vi "Configure Setting Value.vi"(8 "error in (no error)":errorcluster, 9 "Setting Value (0)":dbl min=0.0 step=0.1 format="%^#_6g", 10 "Operation Mode (0: Current)":u16(ring) items=["Current", "Voltage", "Resistance", "Power"], 11 "VISA resource name":refnum<visa-resource-name>) -> (0 "error out":errorcluster, 3 "VISA resource name out":refnum<visa-resource-name>)   [LabVIEW 2021, in "HH PLI Series.lvlib"]
doc: "Sets the operation mode and a static value corresponding to the selected operation mode."
uses:
  HH PLI Series.lvlib
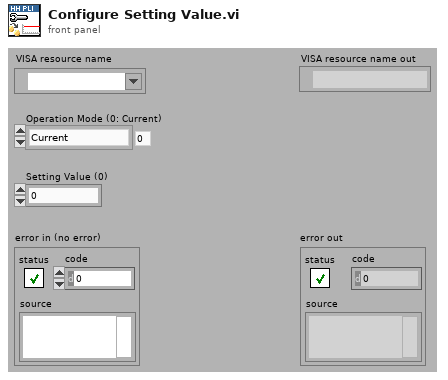
[diagram p1: front panel]
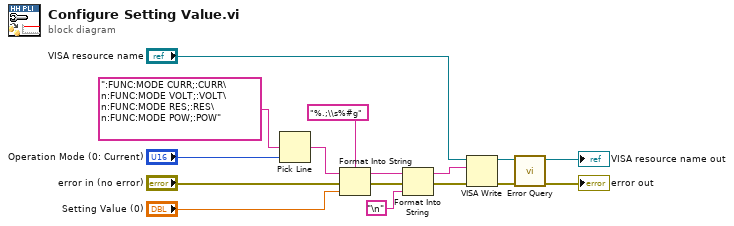
[diagram p0: block diagram]
diagram:
  n1 = Pick Line(multi-line string=":FUNC:MODE CURR;:CURR\n:FUNC:MODE VOLT;:VOLT\n:FUNC:MODE RES;:RES\n:FUNC:MODE POW;:POW", line index="Operation Mode (0: Current)") -> (output string=w6:string)  [unwired: 1 in]
  n2 = Format Into String(format string="%.;\\s%#g", initial string=w6, error in="error in (no error)", "Setting Value (0)") -> (resulting string=w5:string, error out=w2:errorcluster)
  n3 = Format Into String(initial string=w5, error in=w2, "\n") -> (resulting string=w1:string, error out=w4:errorcluster)  [unwired: 1 in]
  n4 = VISA Write(VISA resource name="VISA resource name", write buffer=w1, error in (no error)=w4) -> (VISA resource name out=w10:refnum<visa-resource-name>, error out=w11:errorcluster)  [unwired: 1 out]
  n5 = call "Error Query.vi"("error in (no error)"=w11, "VISA resource name"=w10) -> ("error out"=→"error out":errorcluster, "VISA resource name out"=→"VISA resource name out":refnum<visa-resource-name>)  [unwired: 6 in, 2 out]
